vi "Plotting Convert XY to Waveform.vi"(5 "Macro Filter":bool, 7 "Use Filter?":bool, 8 "Error In":errorcluster, 9 "Plot Name":string, 10 "Y":dbl[](array[numeric]), 11 "X":dbl[](array[numeric])) -> (0 "Error Out":errorcluster, 2 "time stamp":timestamp, 3 "Waveform Graph":waveform(dbl)(graph))   [LabVIEW 2016]
uses:
  <vilib>/Analysis/1siggen.llb/Ramp Pattern by Samples.vi
  <vilib>/gmath/NI_Gmath.lvlib
  <vilib>/Analysis/NI_AALBase.lvlib
panel:
  in  "Use Calculations?":bool
  in  "samples":i32=1000
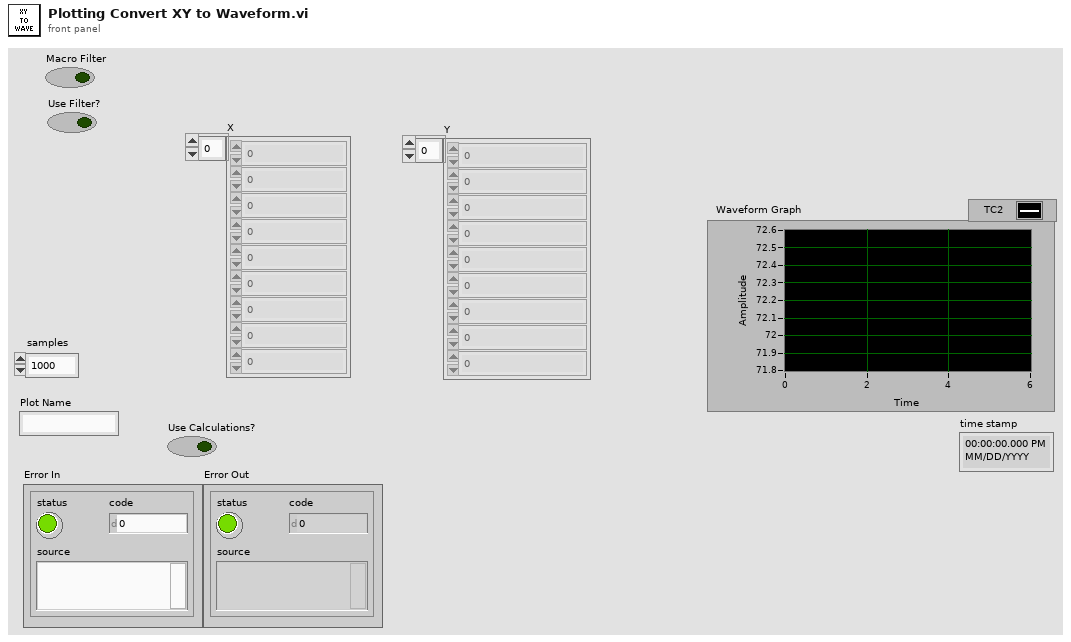
[diagram p1: front panel]
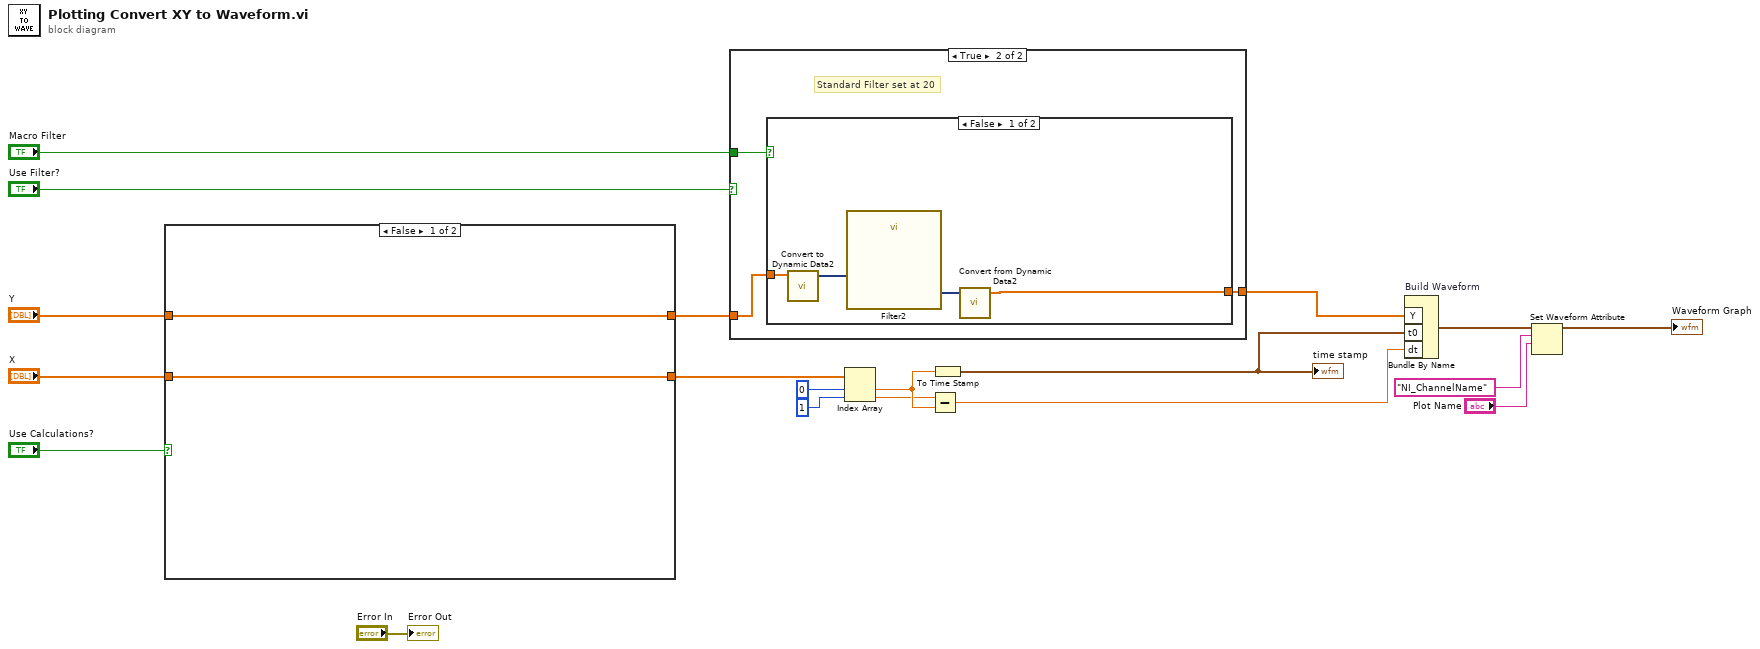
[diagram p0: block diagram]
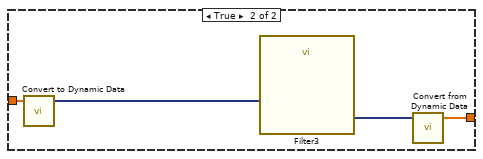
[diagram p3: hidden frame]
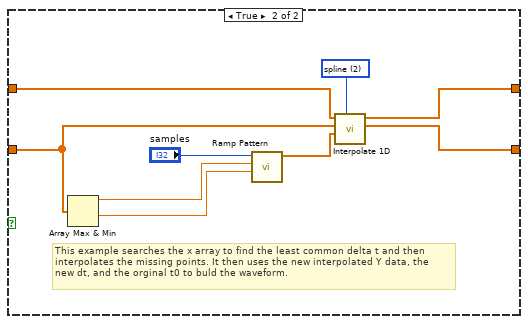
[diagram p4: hidden frame]
diagram:
  n1 = case shown="False" "Use Calculations?" {
    tunnel: "Y" -> [w21 w30]
    tunnel: "X" -> [w20 w29]
    tunnel: [w20 w28] -> w11
    tunnel: [w21 w26] -> w4
    frame False {
    }
    frame True {
      w27 = 2 items=["nearest", "linear", "spline", "cubic Hermite", "Lagrange"] ("method")
      # "This example searches the x array to find the least common delta t and then\ninterpolates the missing points. It then uses the new interpolated Y data, the\nnew dt, and the orginal t0 to buld the waveform."
      n2 = Array Max & Min(array=w29) -> (max value=w22:dbl, min value=w23:dbl)  [unwired: 2 out]
      n3 = call-poly <vilib>:"Ramp Pattern.vi"("start"=w23, "end"=w22, "samples"="samples") -> ("Ramp Pattern"=w25:dbl[])  [unwired: 7 in, 1 out]
      n4 = call <vilib>:"Interpolate 1D.vi"("method"=w27, "xi"=w25, "X"=w29, "Y"=w30) -> ("xi used"=w28:dbl[], "yi"=w26:dbl[])  [unwired: 2 in, 4 out]
    }
  }
  n5 = case shown="True" "Use Filter?" {
    tunnel: w4 -> [w31 w34]
    tunnel: [w31 w33] -> w3
    tunnel: "Macro Filter" -> [_ w32]
    frame False {
    }
    frame True {
      # "Standard Filter set at 20"
      n6 = case shown="False" w32 {
        tunnel: w34 -> [w36 w42]
        tunnel: [w35 w41] -> w33
        frame False {
          n7 = call "Convert to Dynamic Data2"("Array"=w36) -> ("Dynamic Data Type"=w38:dynamicdata)  [unwired: 3 in]
          n8 = call "Filter2"("Signal"=w38) -> ("Filtered Signal"=w37:dynamicdata)  [unwired: 9 in, 1 out]
          n9 = call "Convert from Dynamic Data2"("Dynamic Data Type"=w37) -> ("Array"=w35:dbl[])  [unwired: 3 in]
        }
        frame True {
          n10 = call "Convert to Dynamic Data"("Array"=w42) -> ("Dynamic Data Type"=w39:dynamicdata)  [unwired: 3 in]
          n11 = call "Filter3"("Signal"=w39) -> ("Filtered Signal"=w40:dynamicdata)  [unwired: 9 in, 1 out]
          n12 = call "Convert from Dynamic Data"("Dynamic Data Type"=w40) -> ("Array"=w41:dbl[])  [unwired: 3 in]
        }
      }
    }
  }
  n13 = Index Array "Index Array"(array=w11, index #1=0 ("index"), index #2=1 ("index")) -> (element #1=w13:dbl, element #2=w12:dbl)
  n14 = Subtract(x=w12, y=w13) -> (x-y=w10:dbl)
  n15 = To Time Stamp(1:w13) -> (0:w9:timestamp)
  "time stamp" <- w9
  n16 = Bundle By Name "Build Waveform"("Y"=w3, "t0"=w9, "dt"=w10) -> (w17:waveform(dbl))  [unwired: 1 out]
  n17 = Set Waveform Attribute(5:"Plot Name", 6:"NI_ChannelName" ("name"), 7:w17) -> (3:→"Waveform Graph":waveform(dbl))  [unwired: 1 in, 2 out]
  "Error Out" <- "Error In"
